vi "stop_core (global variable).vi"() -> ()   [LabVIEW 2020, in "core.lvlib"]
uses:
  core.lvlib
panel:
  in  "Stop core?":bool
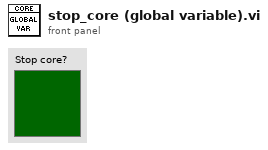
[diagram p1: front panel]
diagram:
